vi "Merge.vi"(8 "error in (no error)":errorcluster, 10 "Field To Merge":refnum<class "Field.lvclass">, 11 "Field In":refnum<class "Field.lvclass">) -> (0 "error out":errorcluster, 3 "Merged Field out":refnum<class "Field.lvclass">)   [LabVIEW 2020, in "Field.lvclass"]
uses:
  Field.lvclass
  Field.lvclass/Field.ctl
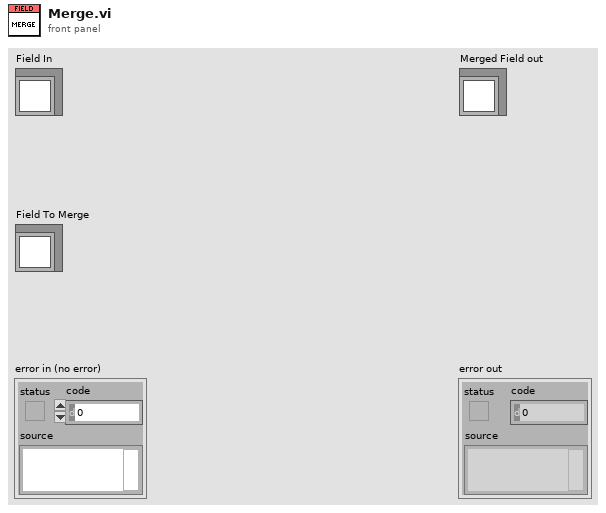
[diagram p1: front panel]
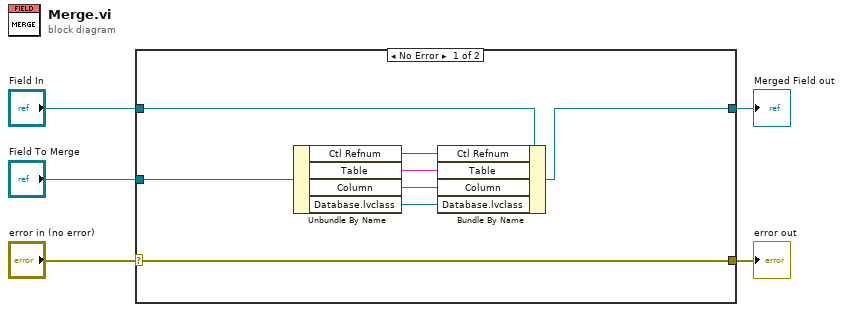
[diagram p0: block diagram]
diagram:
  n1 = case shown="No Error" "error in (no error)" {
    selector: "error in (no error)" -> [w13 w15]
    tunnel: [w13 w15] -> w4
    tunnel: [w11 w14] -> w2
    tunnel: "Field In" -> [w10 w14]
    tunnel: "Field To Merge" -> [w12 _]
    frame No Error {
      n2 = Unbundle By Name(w12) -> ("Ctl Refnum"=w9:refnum<vi>, "Table"=w8:string, "Column"=w7:string, "Database.lvclass"=w6:refnum<class "Database.lvclass">)
      n3 = Bundle By Name(cluster=w10, "Ctl Refnum"=w9, "Table"=w8, "Column"=w7, "Database.lvclass"=w6) -> (w11:refnum<class "Field.lvclass">)
    }
    frame Error {
    }
  }
  "error out" <- w4
  "Merged Field out" <- w2
